vi "Filter 1.vi"(10 "Data for Filtering":T1(array[cluster])) -> (1 "Filtered Data":T1(array[cluster]))   [LabVIEW 2017]
uses:
  <vilib>/Analysis/NI_AALBase.lvlib
panel:
  out "Histogram Graph Ref":T2(graph)
  out "Q3 Ref":dbl format="%.10f"
  out "median Ref":dbl format="%.10f"
  out "Q1 Ref":dbl format="%.10f"
  out "Interquartile Range Ref":dbl
  out "Lower Inner Fence Ref":dbl
  out "Higher Inner Fence Ref":dbl
  out "Reflectivities":dbl[](array[numeric])
  out "Higher Inner Fence":dbl
  out "Lower Inner Fence":dbl
  out "Interquartile Range":dbl
  out "Q1":dbl format="%.10f"
  out "median":dbl format="%.10f"
  out "Q3":dbl format="%.10f"
  out "Histogram Graph":T2(graph)
  out "Distances":dbl[](array[numeric])
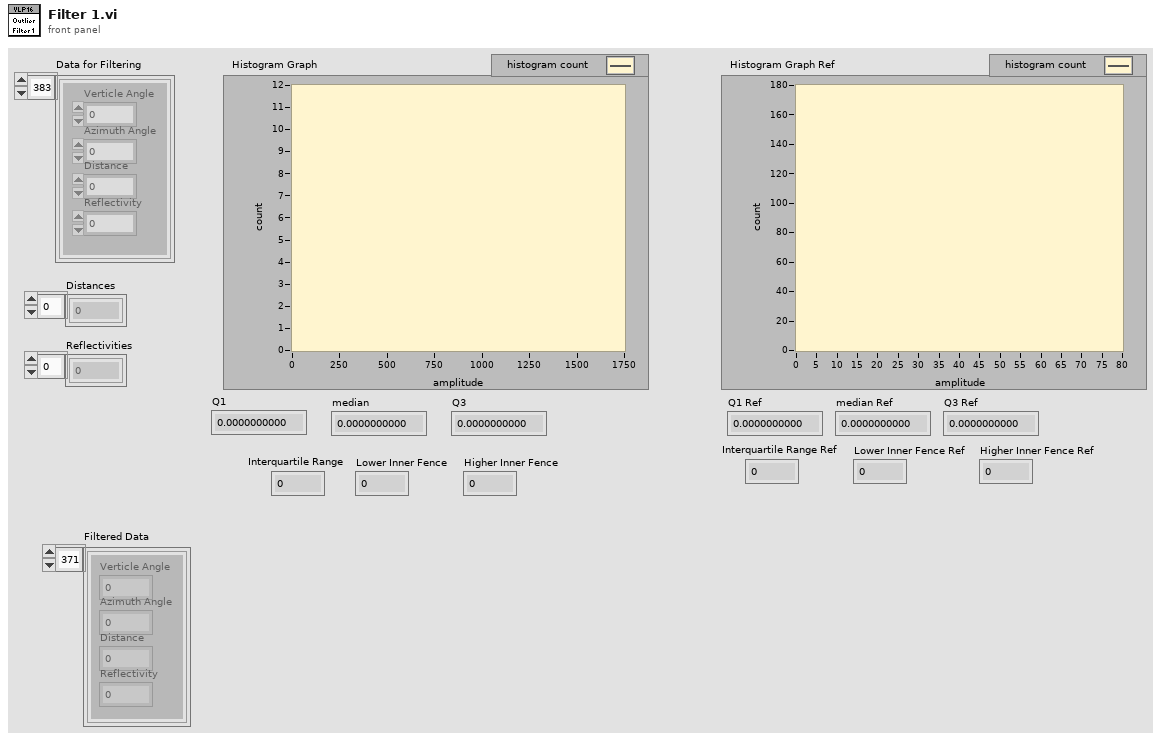
[diagram p1: front panel]
types:
  T1 = cluster{"Verticle Angle":dbl, "Azimuth Angle":dbl, "Distance":dbl, "Reflectivity":dbl}[]
  T2 = cluster{"X Values":dbl[], "Histogram: h(x)":i32[]}
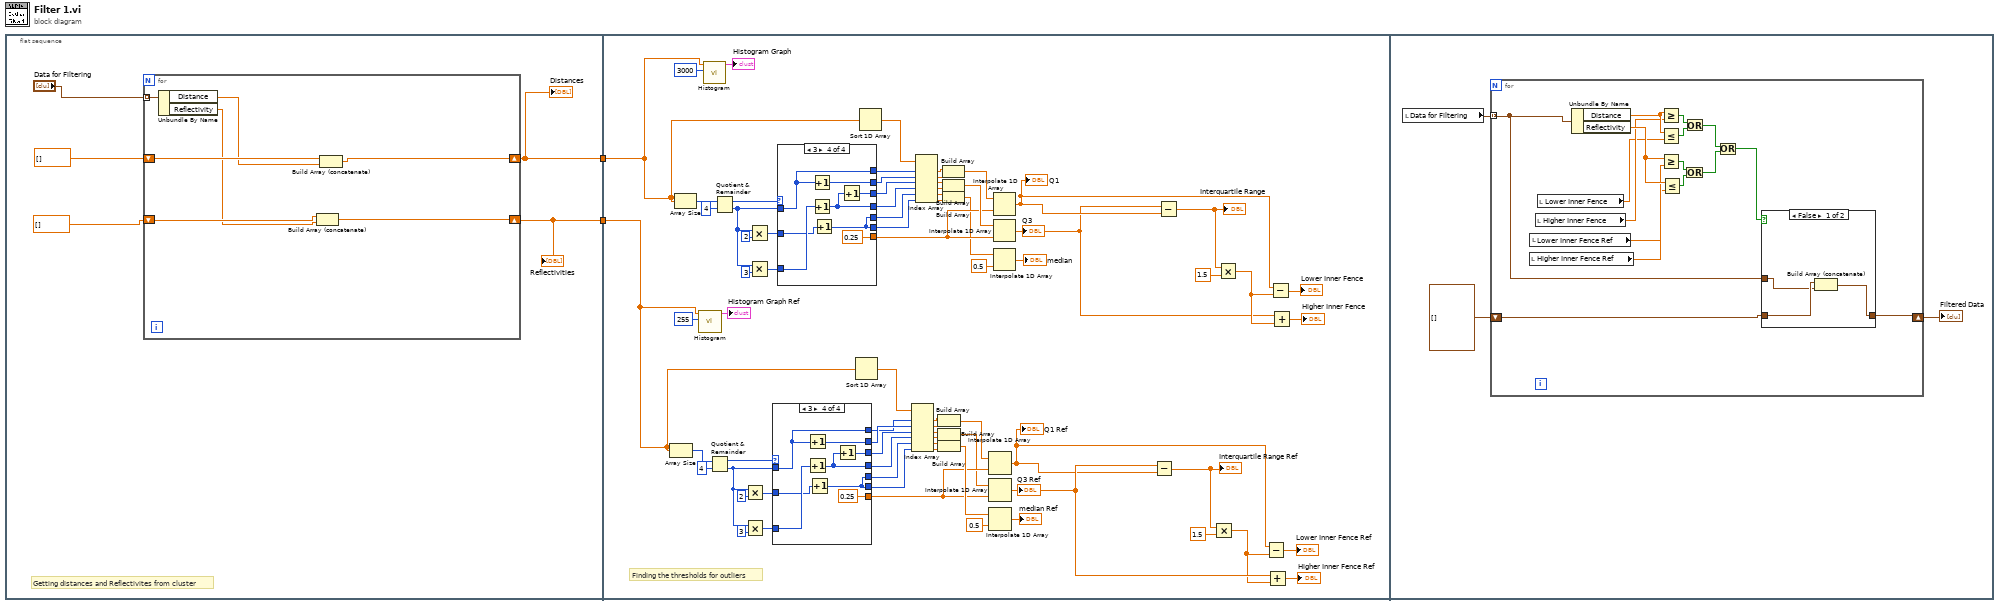
[diagram p0: block diagram]
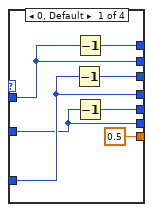
[diagram p2: hidden frame]
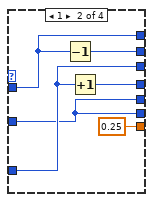
[diagram p3: hidden frame]
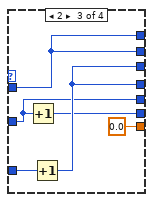
[diagram p4: hidden frame]
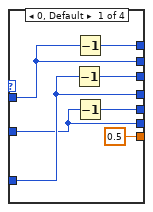
[diagram p5: hidden frame]
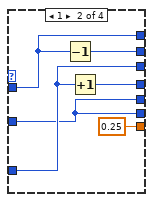
[diagram p6: hidden frame]
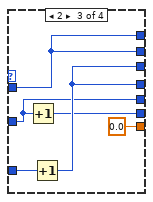
[diagram p7: hidden frame]
diagram:
  n1 = flat-sequence {
    tunnel: [w5] -> w2
    tunnel: [w3] -> w1
    tunnel: w2 -> [w52]
    tunnel: w1 -> [w15]
    frame #0 {
      # "Getting distances and Reflectivites from cluster"
      n2 = for {
        tunnel: "Data for Filtering" -> [w14] mode=indexing
        shift-right: [w12] -> w5
        shift-left: dbl[] [] -> [w13]
        shift-right: [w9] -> w3
        shift-left: dbl[] [] -> [w11]
        n3 = Unbundle By Name(w14) -> ("Distance"=w10:dbl, "Reflectivity"=w8:dbl)
        n4 = Build Array (concatenate)(w11, w8) -> (w9:dbl[])
        n5 = Build Array (concatenate)(w13, w10) -> (w12:dbl[])
      }
      "Distances" <- w5
      "Reflectivities" <- w3
    }
    frame #1 {
      # "Finding the thresholds for outliers"
      n6 = Array Size(array=w15) -> (size(s)=w18:i32)
      n7 = Array Size(array=w52) -> (size(s)=w86:i32)
      n8 = call <vilib>:"Histogram.vi"("intervals"=255, "X"=w15) -> ("Histogram Graph"=→"Histogram Graph Ref":T2)  [unwired: 6 in, 3 out]
      n9 = call <vilib>:"Histogram.vi"("intervals"=3000, "X"=w52) -> ("Histogram Graph"=→"Histogram Graph":T2)  [unwired: 6 in, 3 out]
      n10 = Quotient & Remainder(x=w18, y=4) -> (x-y*floor(x/y)=w20:i32, floor(x/y)=w39:i32)
      n11 = Quotient & Remainder(x=w86, y=4) -> (x-y*floor(x/y)=w84:i32, floor(x/y)=w65:i32)
      n12 = Multiply(x=w39, y=2) -> (x*y=w40:i32)
      n13 = Multiply(x=w39, y=3) -> (x*y=w33:i32)
      n14 = Multiply(x=w65, y=2) -> (x*y=w64:i32)
      n15 = Multiply(x=w65, y=3) -> (x*y=w71:i32)
      n16 = case shown="3" w20 {
        tunnel: w39 -> [w95 w100 w107 w114]
        tunnel: [w93 w100 w107 w114] -> w28
        tunnel: [w95 w97 w107 w115] -> w29
        tunnel: [w91 w99 w104 w112] -> w30
        tunnel: [w94 w98 w104 w110] -> w31
        tunnel: w33 -> [w94 w99 w106 w111]
        tunnel: [0.5 0.25 0.0 0.25] -> w34
        tunnel: w40 -> [w89 w96 w103 w109]
        tunnel: [w90 w96 w103 w108] -> w42
        tunnel: [w89 w96 w102 w108] -> w43
        frame 0, Default {
          n17 = Decrement(x=w94) -> (x-1=w91:i32)
          n18 = Decrement(x=w95) -> (x-1=w93:i32)
          n19 = Decrement(x=w89) -> (x-1=w90:i32)
        }
        frame 1 {
          n20 = Decrement(x=w100) -> (x-1=w97:i32)
          n21 = Increment(x=w99) -> (x+1=w98:i32)
        }
        frame 2 {
          n22 = Increment(x=w103) -> (x+1=w102:i32)
          n23 = Increment(x=w106) -> (x+1=w104:i32)
        }
        frame 3 {
          n24 = Increment(x=w114) -> (x+1=w115:i32)
          n25 = Increment(x=w111) -> (x+1=w110:i32)
          n26 = Increment(x=w109) -> (x+1=w108:i32)
          n27 = Increment(x=w110) -> (x+1=w112:i32)
        }
      }
      n28 = case shown="3" w84 {
        tunnel: w65 -> [w122 w127 w134 w141]
        tunnel: [w120 w127 w134 w141] -> w76
        tunnel: [w122 w124 w134 w142] -> w75
        tunnel: [w118 w126 w131 w139] -> w74
        tunnel: [w121 w125 w131 w137] -> w73
        tunnel: w71 -> [w121 w126 w133 w138]
        tunnel: [0.5 0.25 0.0 0.25] -> w70
        tunnel: w64 -> [w116 w123 w130 w136]
        tunnel: [w117 w123 w130 w135] -> w62
        tunnel: [w116 w123 w129 w135] -> w61
        frame 0, Default {
          n29 = Decrement(x=w121) -> (x-1=w118:i32)
          n30 = Decrement(x=w122) -> (x-1=w120:i32)
          n31 = Decrement(x=w116) -> (x-1=w117:i32)
        }
        frame 1 {
          n32 = Decrement(x=w127) -> (x-1=w124:i32)
          n33 = Increment(x=w126) -> (x+1=w125:i32)
        }
        frame 2 {
          n34 = Increment(x=w130) -> (x+1=w129:i32)
          n35 = Increment(x=w133) -> (x+1=w131:i32)
        }
        frame 3 {
          n36 = Increment(x=w141) -> (x+1=w142:i32)
          n37 = Increment(x=w138) -> (x+1=w137:i32)
          n38 = Increment(x=w136) -> (x+1=w135:i32)
          n39 = Increment(x=w137) -> (x+1=w139:i32)
        }
      }
      n40 = Sort 1D Array(array=w15) -> (sorted array=w21:dbl[])
      n41 = Sort 1D Array(array=w52) -> (sorted array=w83:dbl[])
      n42 = Index Array(array=w21, index #1=w28, index #2=w29, index #3=w30, index #4=w31, index #5=w42, index #6=w43) -> (element #1=w22:dbl, element #2=w23:dbl, element #3=w24:dbl, element #4=w25:dbl, element #5=w35:dbl, element #6=w36:dbl)
      n43 = Index Array(array=w83, index #1=w76, index #2=w75, index #3=w74, index #4=w73, index #5=w62, index #6=w61) -> (element #1=w82:dbl, element #2=w81:dbl, element #3=w80:dbl, element #4=w79:dbl, element #5=w69:dbl, element #6=w68:dbl)
      n44 = Build Array(w22, w23) -> (w26:dbl[])
      n45 = Build Array(w24, w25) -> (w27:dbl[])
      n46 = Build Array(w35, w36) -> (w37:dbl[])
      n47 = Build Array(w82, w81) -> (w78:dbl[])
      n48 = Build Array(w80, w79) -> (w77:dbl[])
      n49 = Build Array(w69, w68) -> (w67:dbl[])
      n50 = Interpolate 1D Array(1:w34, 2:w26) -> (0:w49:dbl)
      "Q1 Ref" <- w49
      n51 = Interpolate 1D Array(1:w34, 2:w27) -> (0:w50:dbl)
      "Q3 Ref" <- w50
      n52 = Interpolate 1D Array(1:0.5 ("fractional index or x"), 2:w37) -> (0:→"median Ref":dbl)
      n53 = Interpolate 1D Array(1:w70, 2:w78) -> (0:w55:dbl)
      "Q1" <- w55
      n54 = Interpolate 1D Array(1:w70, 2:w77) -> (0:w54:dbl)
      "Q3" <- w54
      n55 = Interpolate 1D Array(1:0.5 ("fractional index or x"), 2:w67) -> (0:→"median":dbl)
      n56 = Subtract(x=w50, y=w49) -> (x-y=w51:dbl)
      "Interquartile Range Ref" <- w51
      n57 = Subtract(x=w54, y=w55) -> (x-y=w53:dbl)
      "Interquartile Range" <- w53
      n58 = Multiply(x=w51, y=1.5) -> (x*y=w46:dbl)
      n59 = Multiply(x=w53, y=1.5) -> (x*y=w58:dbl)
      n60 = Subtract(x=w49, y=w46) -> (x-y=→"Lower Inner Fence Ref":dbl)
      n61 = Add(x=w50, y=w46) -> (x+y=→"Higher Inner Fence Ref":dbl)
      n62 = Subtract(x=w55, y=w58) -> (x-y=→"Lower Inner Fence":dbl)
      n63 = Add(x=w54, y=w58) -> (x+y=→"Higher Inner Fence":dbl)
    }
    frame #2 {
      n64 = local read "Data for Filtering"() -> (w144:T1)
      n65 = for {
        shift-right: [w148] -> w143
        shift-left: cluster{dbl, dbl, dbl, dbl}[] [] -> [w149]
        tunnel: w144 -> [w146] mode=indexing
        n66 = local read "Higher Inner Fence Ref"() -> (w151:dbl)
        n67 = local read "Lower Inner Fence Ref"() -> (w150:dbl)
        n68 = local read "Higher Inner Fence"() -> (w153:dbl)
        n69 = local read "Lower Inner Fence"() -> (w152:dbl)
        n70 = Unbundle By Name(w146) -> ("Distance"=w155:dbl, "Reflectivity"=w154:dbl)
        n71 = Greater Or Equal?(x=w155, y=w153) -> (x >= y?=w159:bool)
        n72 = Less Or Equal?(x=w155, y=w152) -> (x <= y?=w161:bool)
        n73 = Greater Or Equal?(x=w154, y=w151) -> (x >= y?=w160:bool)
        n74 = Less Or Equal?(x=w154, y=w150) -> (x <= y?=w158:bool)
        n75 = Or(x=w160, y=w158) -> (x .or. y?=w156:bool)
        n76 = Or(x=w159, y=w161) -> (x .or. y?=w157:bool)
        n77 = Or(x=w157, y=w156) -> (x .or. y?=w147:bool)
        n78 = case shown="False" w147 {
          tunnel: w149 -> [w164 w165]
          tunnel: [w162 w165] -> w148
          tunnel: w146 -> [w163 _]
          frame False {
            n79 = Build Array (concatenate)(w164, w163) -> (w162:T1)
          }
          frame True {
          }
        }
      }
      "Filtered Data" <- w143
    }
  }
